vi "Set Exposure.vi"(8 "error in":errorcluster, 11 "DMK33UP2000 in":refnum<class "DMK33UP2000.lvclass">) -> (0 "error out":errorcluster, 2 "Supported?":bool, 3 "DMK33UP2000 out":refnum<class "DMK33UP2000.lvclass">)   [LabVIEW 2018, in "DMK33UP2000.lvlib" / "DMK33UP2000.lvclass"]
uses:
  DMK33UP2000.lvclass
  builds/Camera.lvlibp/Camera.lvclass
  <resource>/objmgr/imaqdx.rc
  C:/Users/Ron.Dexter.LUMINARTECH/Desktop/builds/Camera.lvlibp/Camera.lvclass
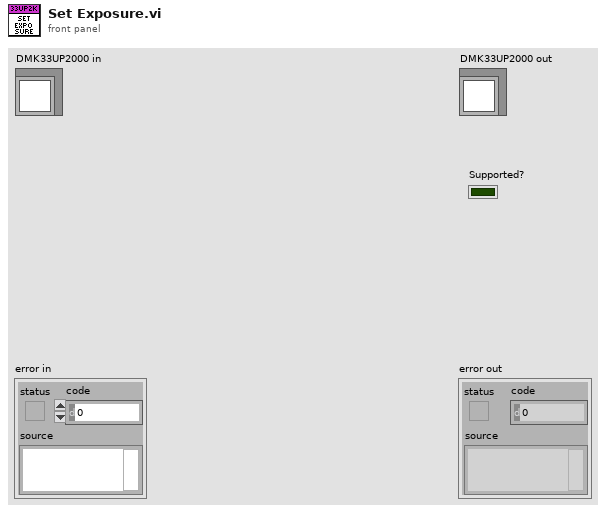
[diagram p1: front panel]
types:
  T1 = typedef "Camera.lvlibp/IMAQdx.ctl" = refnum<k21>
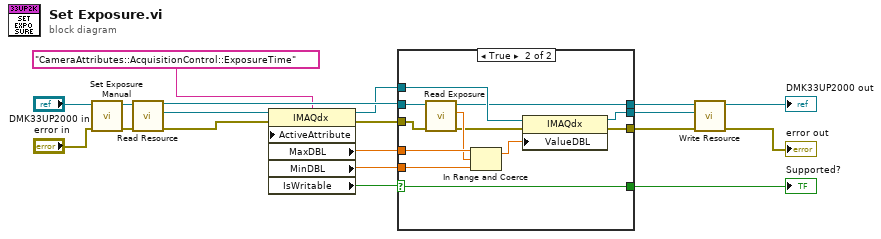
[diagram p0: block diagram]
diagram:
  n1 = call "Set Exposure Manual.vi"("error in"="error in", "DMK33UP2000 in"="DMK33UP2000 in") -> ("error out"=w2:errorcluster, "DMK33UP2000 out"=w1:refnum<class "DMK33UP2000.lvclass">)  [unwired: 7 in, 1 out]
  n2 = call "Read Resource.vi"("error in (no error)"=w2, "Camera in"=w1) -> ("error out"=w10:errorcluster, "IMAQdx Session"=w9:T1, "Camera out"=w14:refnum<class "DMK33UP2000.lvclass">)  [unwired: 7 in]
  n3 = property class="IMAQdx"(reference=w9, error in=w10, "ActiveAttribute"="CameraAttributes::AcquisitionControl::ExposureTime") -> (reference out=w12:T1, error out=w16:errorcluster, "MaxDBL"=w18:dbl, "MinDBL"=w19:dbl, "IsWritable"=w11:bool)
  n4 = case shown="True" w11 {
    selector: w11 -> [w21 w35]
    tunnel: [w21 w35] -> w5
    tunnel: w12 -> [w22 w34]
    tunnel: [w22 w33] -> w13
    tunnel: w14 -> [w23 w28]
    tunnel: [w23 w24] -> w15
    tunnel: w16 -> [w20 w27]
    tunnel: [w20 w32] -> w17
    tunnel: w18 -> [_ w31]
    tunnel: w19 -> [_ w30]
    frame False {
    }
    frame True {
      n5 = call "Read Exposure.vi"("error in (no error)"=w27, "Camera in"=w28) -> ("error out"=w25:errorcluster, "Exposure"=w26:dbl, "Camera out"=w24:refnum<class "DMK33UP2000.lvclass">)  [unwired: 7 in]
      n6 = In Range and Coerce(upper limit=w31, x=w26, lower limit=w30) -> (coerced(x)=w29:dbl)  [unwired: 1 out]
      n7 = property class="IMAQdx"(reference=w34, error in=w25, "ValueDBL"=w29) -> (reference out=w33:T1, error out=w32:errorcluster)
    }
  }
  "Supported?" <- w5
  n8 = call "Write Resource.vi"("error in (no error)"=w17, "IMAQdx Session"=w13, "Camera in"=w15) -> ("error out"=→"error out":errorcluster, "Camera out"=→"DMK33UP2000 out":refnum<class "DMK33UP2000.lvclass">)  [unwired: 7 in]
